vi "PublisherExample.vi"() -> ()   [LabVIEW 2016]
doc: "Sample publisher. Publishers a string to the topic chatter"
uses:
  ROS/Code/Console/Servers/ServerSubs/TopicDef.ctl
  ROS/Code/SubVIs/_ROSDirection.ctl
  ROS/MessageBuilding/std_msgs/subs/stringScalar.vi
  ROS/Code/_ROSDefinition.vi
panel:
  in  "stop":bool
  out "error out":errorcluster
  in  "I said:":string="Hello world!"
  # "Instructions:\n1. Run Publisher example\n2. Run Subscriber eample"
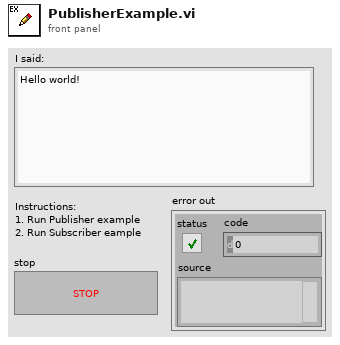
[diagram p1: front panel]
types:
  T1 = typedef "TopicDef.ctl" = cluster{"Topic":string, "Type":string, "Action":T2, "Update (ms)":u16, "queue size":u16}
  T2 = typedef "_ROSDirection.ctl" = enum16{"Node", "Publisher", "Subscriber", "ServiceClient", "ServiceProvider"}
  T3 = typedef "_ROSControl.ctl" = cluster{"topic port":u16, "Node":string, "topic":string, "type":string, "node port":u16, "error ":errorcluster, "Direction":T2, "Update (ms)":u16, "FIFO size":u16}
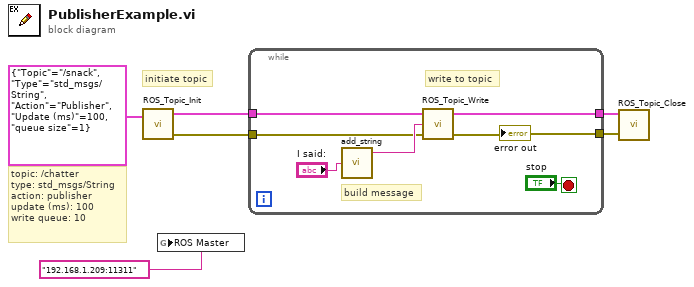
[diagram p0: block diagram]
diagram:
  # "initiate topic"
  # "topic: /chatter\ntype: std_msgs/String\naction: publisher\nupdate (ms): 100\nwrite queue: 10"
  n1 = call "ROS_Topic_Init.vi"("Definitions"=T1 {"Topic"="/snack", "Type"="std_msgs/String", "Action"=enum."Publisher", "Update (ms)"=100, "queue size"=1}) -> ("ROS out"=w5:T3, "error out"=w4:errorcluster)  [unwired: 2 in]
  n2 = global write "_ROSDefinition.vi" "ROS Master"("192.168.1.209:11311" ("ROS Master")) -> ()
  n3 = while {
    tunnel: w5 -> [w13]
    tunnel: w4 -> [w10]
    tunnel: [w8] -> w3
    tunnel: [w7] -> w2
    stop <- "stop" stop-if-true
    # "build message"
    # "write to topic"
    n4 = call-poly "add_string.vi"("String"="I said:") -> ("msg out"=w11:string)  [unwired: 4 in]
    n5 = call "ROS_Topic_Write.vi"("error in (no error)"=w10, "Msg in"=w11, "ROS in"=w13) -> ("error out"=w7:errorcluster, "ROS out"=w8:T3)  [unwired: 1 in]
    "error out" <- w7
  }
  n6 = call "ROS_Topic_Close.vi"("error in"=w2, "ROS in"=w3) -> ()  [unwired: 2 in, 1 out]
